vi "Stop.vi"(8 "error in (no error)":errorcluster, 11 "Sound Player in":refnum<class "Sound Player.lvclass">) -> (0 "error out":errorcluster, 3 "Sound Player out":refnum<class "Sound Player.lvclass">)   [LabVIEW 2017, in "Sound Player.lvclass"]
doc: "Stop any sounds currently playing on the device, but do not actually shut down the sound player. Further calls to Play on this device should continue to work.\n\nThis method is not actually used in the Sound Demo application, but it is included for completeness and future expansion."
uses:
  Sound Player.lvclass
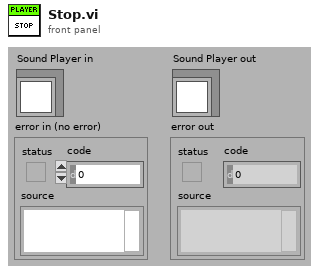
[diagram p1: front panel]
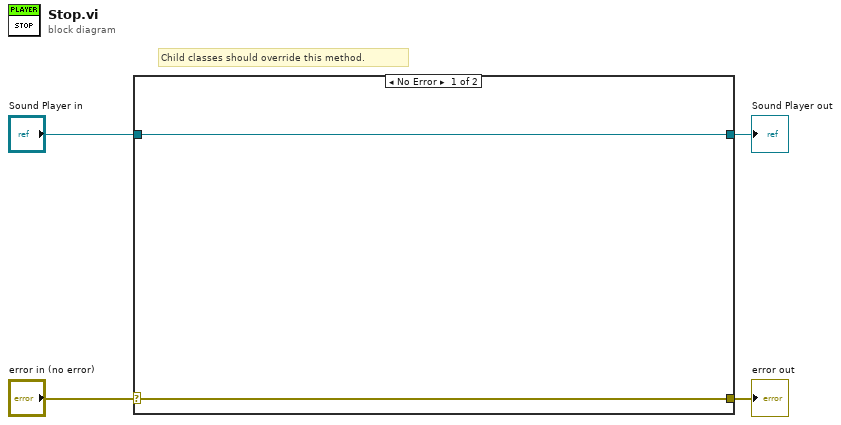
[diagram p0: block diagram]
diagram:
  # "Child classes should override this method."
  n1 = case shown="No Error" "error in (no error)" {
    selector: "error in (no error)" -> [w5 w8]
    tunnel: [w5 w8] -> w3
    tunnel: [w6 w7] -> w1
    tunnel: "Sound Player in" -> [w6 w7]
    frame No Error {
    }
    frame Error {
    }
  }
  "error out" <- w3
  "Sound Player out" <- w1
